vi "FPGAPowerMeasurement.vi"() -> ()   [LabVIEW 2009]
panel:
  in  "stop":bool
  out "Total Power Consumption":dbl
  out "Waveform Graph 3":dynamicdata(graph)
  out "Power Consumption":dynamicdata(graph)
  out "Voltage":dynamicdata(graph) caption="data"
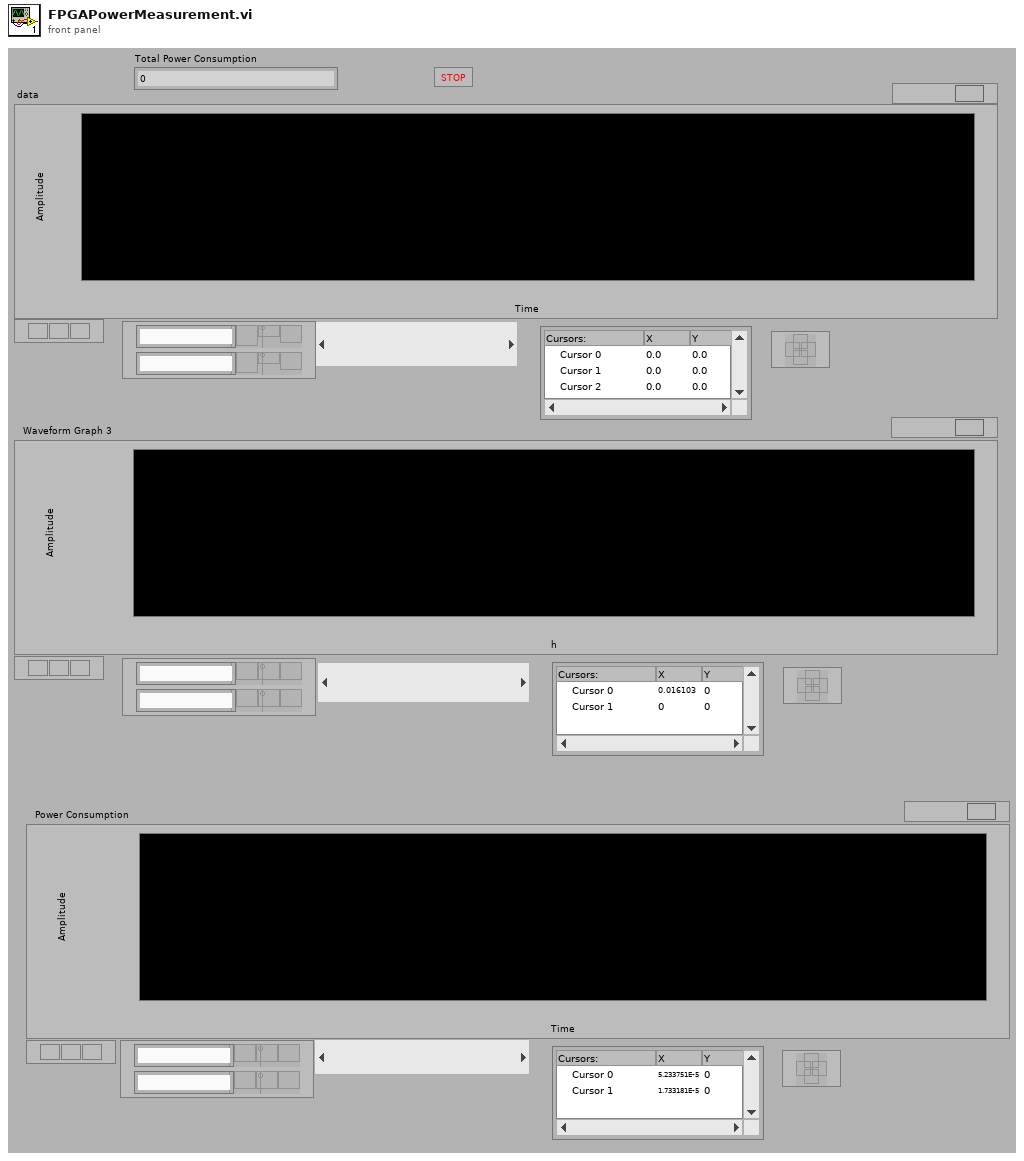
[diagram p1: front panel]
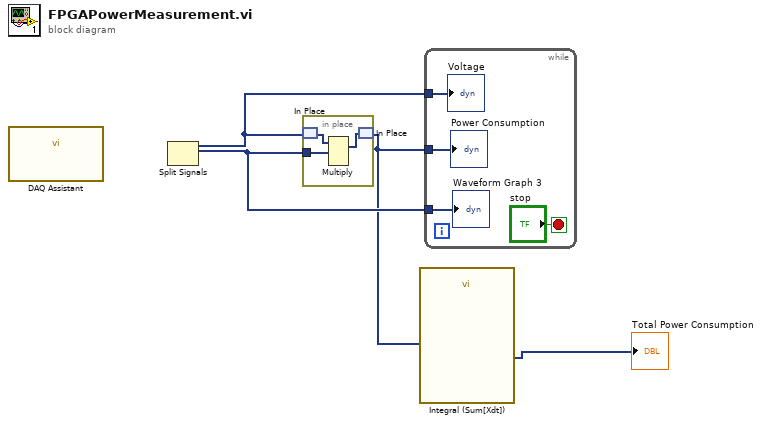
[diagram p0: block diagram]
diagram:
  n1 = call "DAQ Assistant"() -> ()  [unwired: 20 in]
  n2 = Split Signals() -> (w3:dynamicdata, w4:dynamicdata)  [unwired: 1 in, 4 out]
  n3 = in-place {
    in-place-border: w4 -> [w7]
    n4 = in-place-match #1(w3) -> (w6:dynamicdata)
    n5 = Multiply(1:w7, 2:w6) -> (0:w5:dynamicdata)  [unwired: 1 in, 1 out]
    n6 = in-place-match #1(w5) -> (w2:dynamicdata)
  }
  n7 = call "Integral (Sum[Xdt])"("Signals"=w2) -> ("Result"=→"Total Power Consumption":dynamicdata)  [unwired: 1 in, 5 out]
  n8 = while {
    tunnel: w4 -> [w11]
    tunnel: w3 -> [w10]
    tunnel: w2 -> [w9]
    stop <- "stop" stop-if-true
    "Voltage" <- w10
    "Power Consumption" <- w9
    "Waveform Graph 3" <- w11
  }
